vi "MSScript_Exe_MSProcess.vi"(8 "error in (no error)":errorcluster, 9 "EXPR Index in":i32, 11 "MSScript in":refnum<class "MSScript.lvclass">) -> (0 "error out":errorcluster, 1 "EXPR Index out":i32, 3 "MSScript out":refnum<class "MSScript.lvclass">)   [LabVIEW 2018, in "MSScript.lvclass"]
uses:
  MSScript.lvclass
  MSScript.lvclass/MSScript.ctl
  MSScript_Error_(6006)ParamErr.vi
  MSScript_Error_(6002)UndefinedSentence.vi
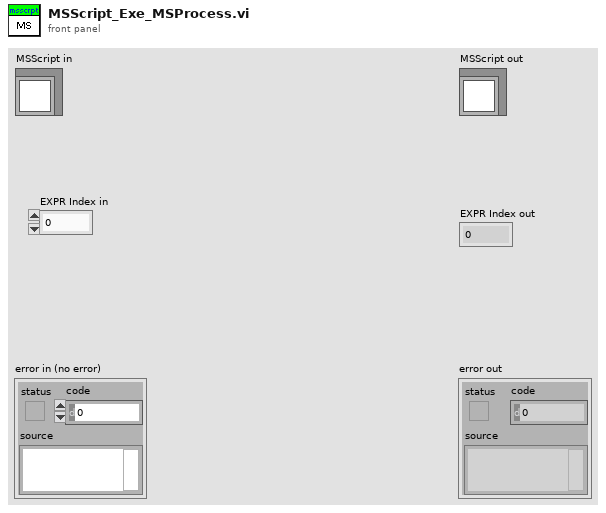
[diagram p1: front panel]
types:
  T1 = cluster{"Colour":u32, "Italic":bool, "Bold":bool}
  T2 = cluster{"Type":string, "NAME":cluster{"STR":string, "Start":i32}, "PARAMs":cluster{"STR":string, "Start":i32}[]}[]
  T3 = cluster{"Type":string, "NAME":cluster{"STR":string, "Start":i32}, "PARAMs":cluster{"STR":string, "Start":i32}[]}
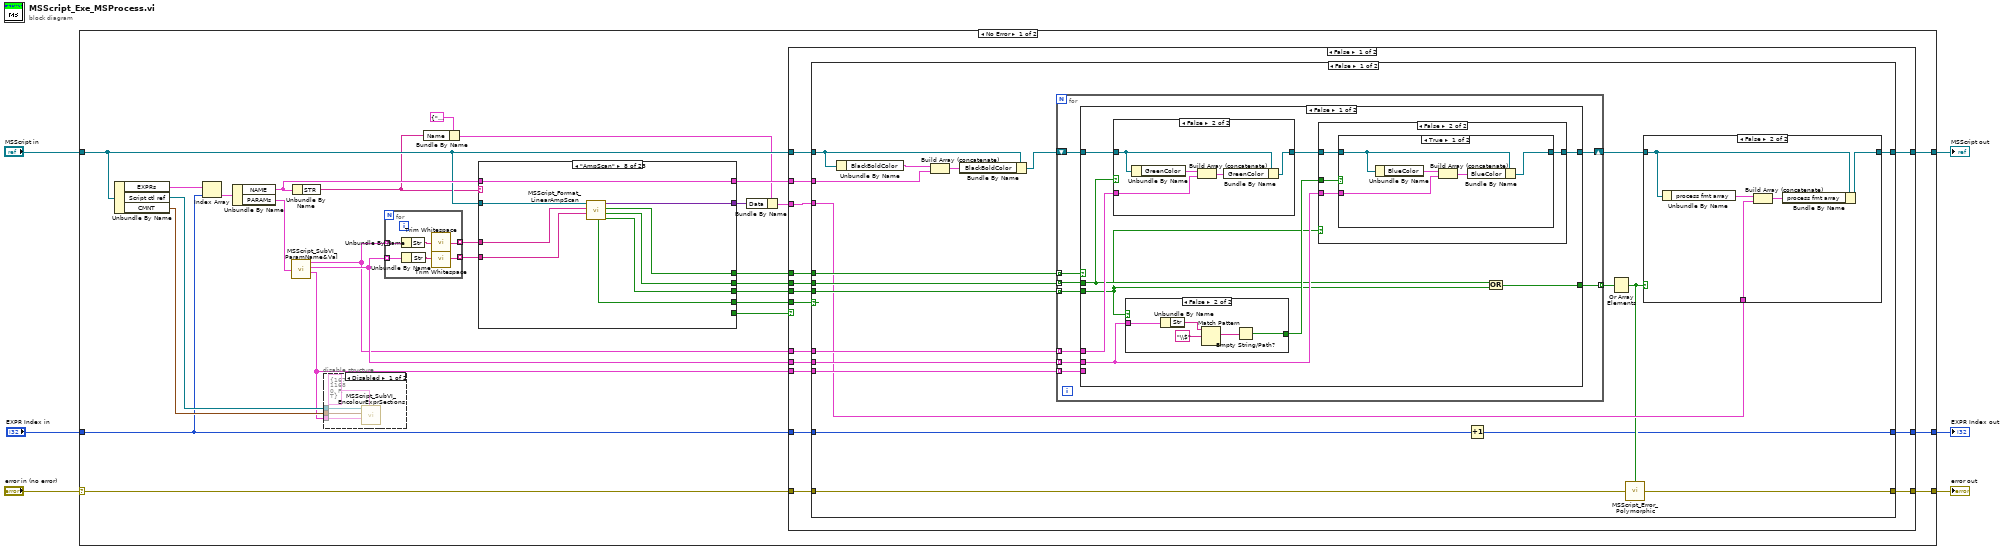
[diagram p0: block diagram]
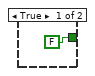
[diagram p3: hidden frame]
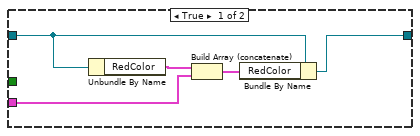
[diagram p4: hidden frame]
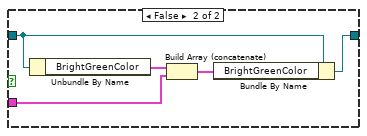
[diagram p5: hidden frame]
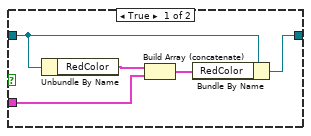
[diagram p6: hidden frame]
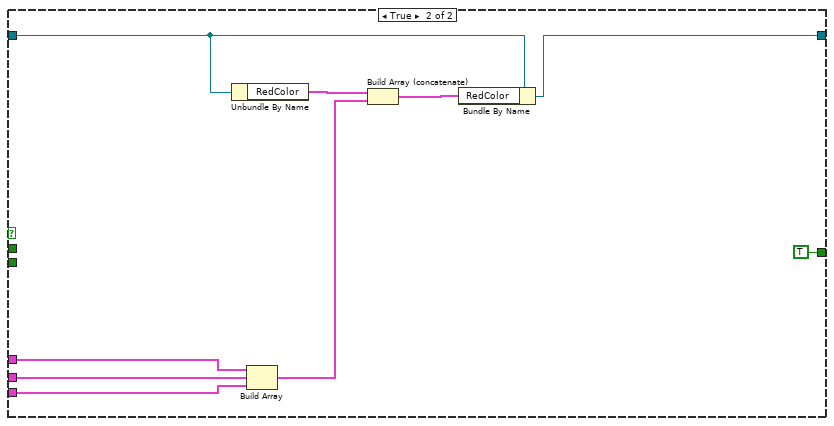
[diagram p7: hidden frame]
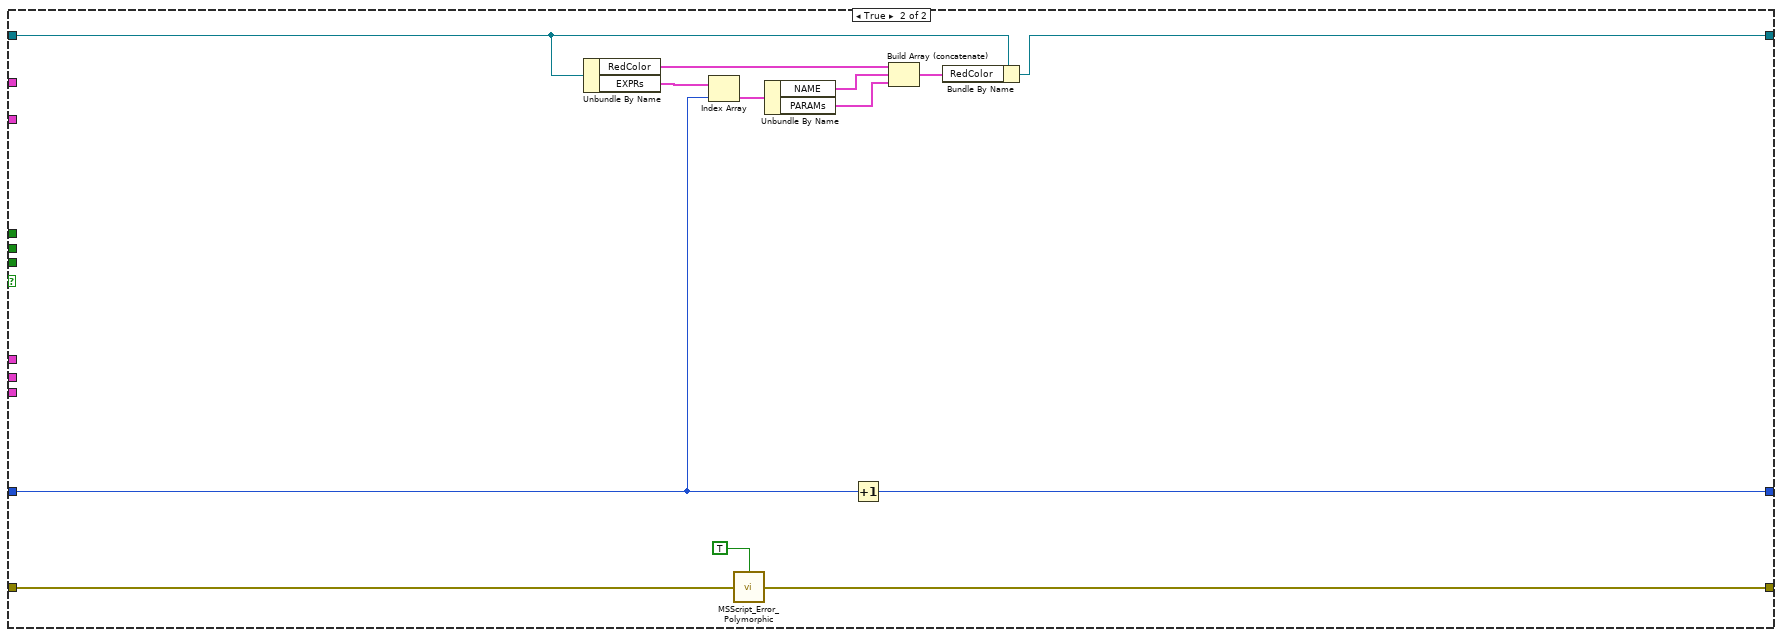
[diagram p8: hidden frame]
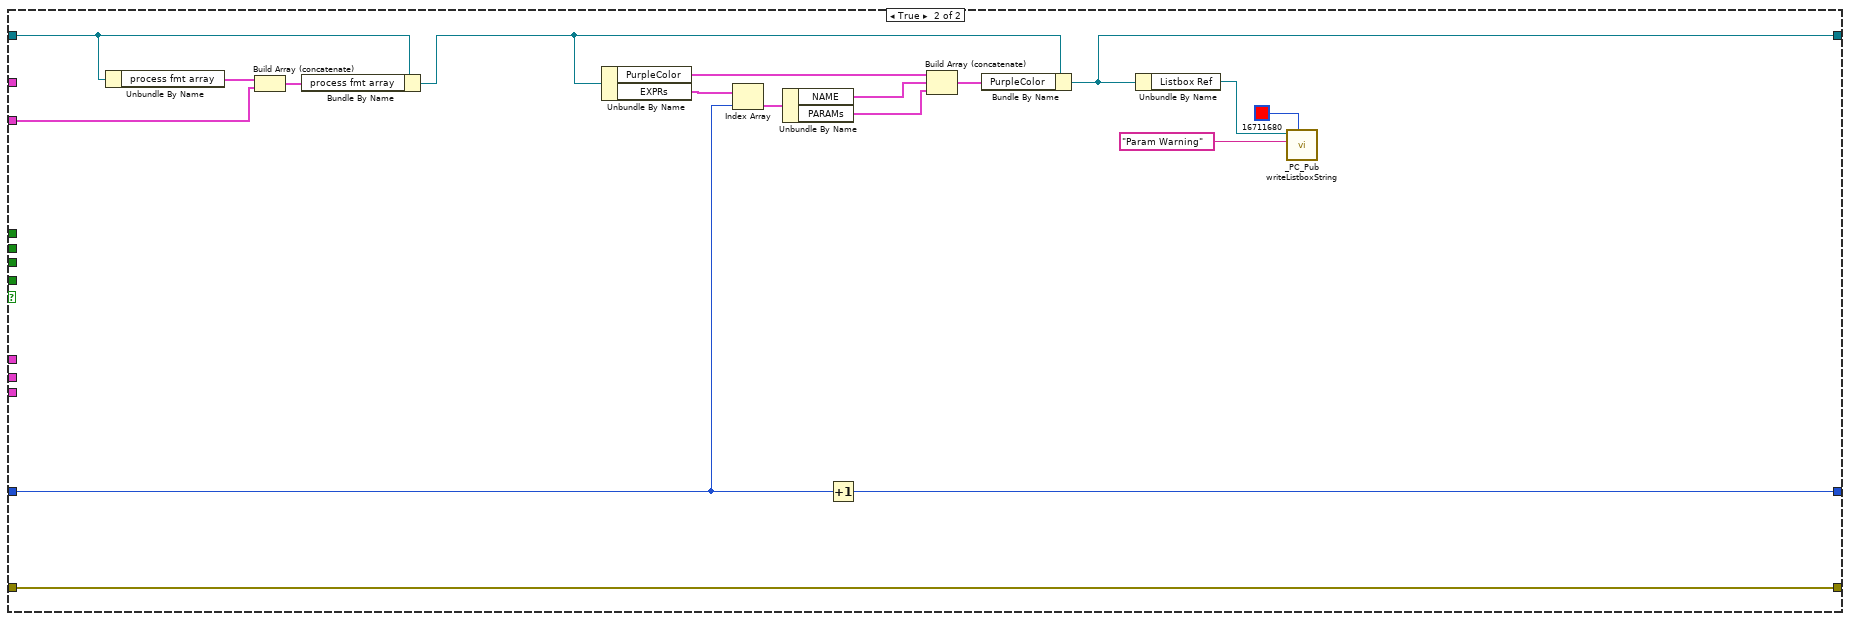
[diagram p9: hidden frame]
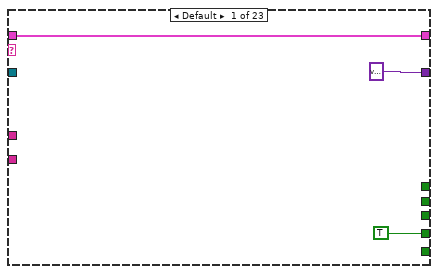
[diagram p11: hidden frame]
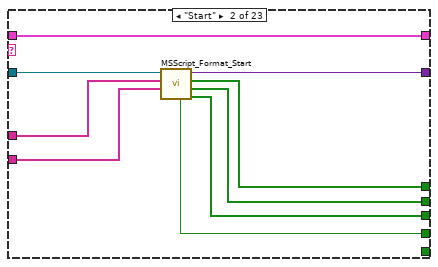
[diagram p12: hidden frame]
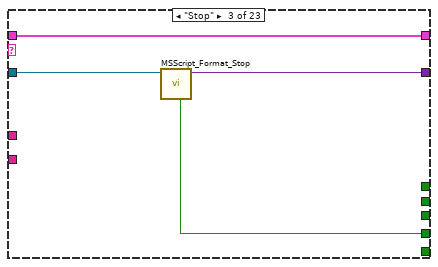
[diagram p13: hidden frame]
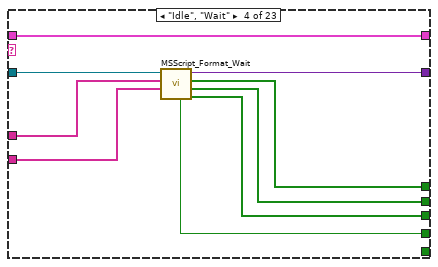
[diagram p14: hidden frame]
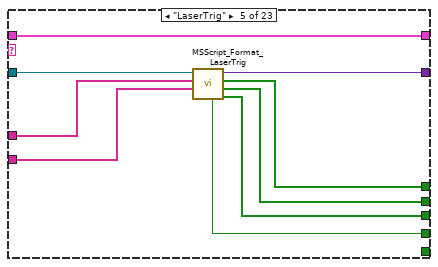
[diagram p15: hidden frame]
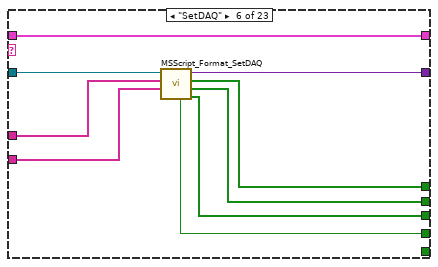
[diagram p16: hidden frame]
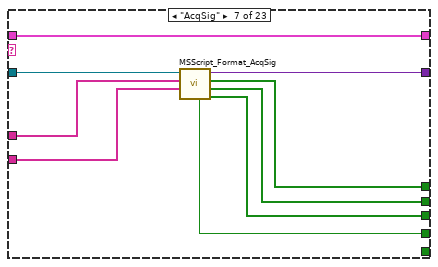
[diagram p17: hidden frame]
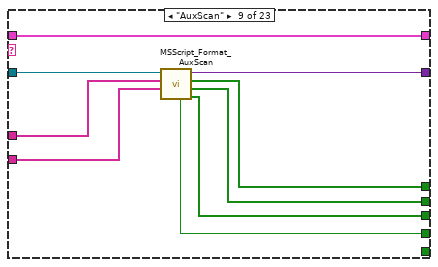
[diagram p18: hidden frame]
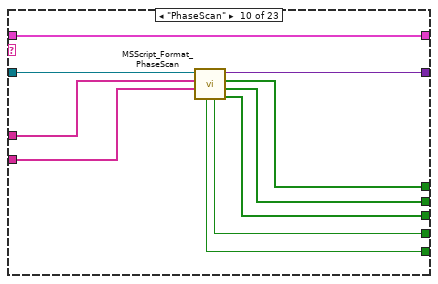
[diagram p19: hidden frame]
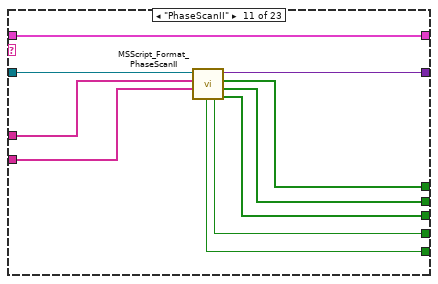
[diagram p20: hidden frame]
diagram:
  n1 = case shown="No Error" "error in (no error)" {
    selector: "error in (no error)" -> [w22 w379]
    tunnel: [w21 w379] -> w5
    tunnel: [w24 w378] -> w3
    tunnel: "MSScript in" -> [w14 w378]
    tunnel: "EXPR Index in" -> [w20 _]
    tunnel: [w16 _] -> w1
    frame No Error {
      n2 = Unbundle By Name(w14) -> ("EXPRs"=w34:T2, "Script ctl ref"=w30:refnum<vi>, "CMNT"=w31:cluster{"Start":u32, "End":u32}[])
      n3 = Index Array(array=w34, index=w20) -> (element=w33:T3)
      n4 = Unbundle By Name(w33) -> ("NAME"=w15:cluster{"STR":string, "Start":i32}, "PARAMs"=w32:cluster{"STR":string, "Start":i32}[])
      n5 = call "MSScript_SubVI_ParamName&Val.vi"("PARAMs"=w32) -> ("PARAM.NAMEs"=w18:cluster{"Str":string, "Start":i32}[], "PARAM.VALs"=w19:cluster{"Str":string, "Start":i32}[], "PARAM.EqualSign"=w17:cluster{"Str":string, "Start":i32}[])  [unwired: 4 in, 1 out]
      n6 = Unbundle By Name(w15) -> ("STR"=w11:string)
      n7 = disable-structure shown="Disabled" {
        disable-tunnel: w31 -> [w172 _]
        disable-tunnel: w30 -> [w171 _]
        disable-tunnel: w17 -> [w170 _]
        frame Disabled {
          n8 = call "MSScript_SubVI_EncolourExprSections.vi"("TextProperties"=T1 {"Colour"=16711680, "Italic"=FALSE, "Bold"=TRUE}, "Expression Sections"=w170, "CMNT"=w172, "String in"=w171) -> ()  [unwired: 7 in, 1 out]
        }
        frame Enabled {
        }
      }
      n9 = for {
        tunnel: w18 -> [w178] mode=indexing
        tunnel: w19 -> [w177] mode=indexing
        tunnel: [w174] -> w29 mode=indexing
        tunnel: [w173] -> w28 mode=indexing
        n10 = Unbundle By Name(w178) -> ("Str"=w176:string)
        n11 = Unbundle By Name(w177) -> ("Str"=w175:string)
        n12 = call <vilib>:"Trim Whitespace.vi"("string"=w176) -> ("trimmed string"=w174:string)  [unwired: 1 in]
        n13 = call <vilib>:"Trim Whitespace.vi"("string"=w175) -> ("trimmed string"=w173:string)  [unwired: 1 in]
      }
      n14 = Bundle By Name(cluster=cluster{"Name":string, "Data":variant} {"Name"="", "Data"=variant} ("process fmt"), "Name"=w11) -> (w9:cluster{"Name":string, "Data":variant})
      n15 = case shown="\"AmpScan\"" w11 {
        tunnel: w29 -> [_ w188 _ w203 w207 w216 w223 w239 w243 w258 w260 w270 w280 w291 w305 w314 w323 w332 w338 w348 w353 w368 w377]
        tunnel: w28 -> [_ w187 _ w202 w208 w215 w222 w238 w242 w257 w261 w271 w281 w290 w304 w313 w322 w331 w337 w347 w352 w367 w376]
        tunnel: [variant w190 w194 w197 w212 w221 w228 w237 w248 w256 w267 w277 w286 w296 w303 w312 w317 w324 w339 w346 w358 w362 w371] -> w8
        tunnel: [_ w189 _ w198 w211 w220 w227 w236 w246 w255 w266 w276 w285 w292 w302 w311 w318 w327 w333 w345 w357 w363 w372] -> w27
        tunnel: [_ w186 _ w199 w210 w219 w226 w235 w245 w254 w265 w275 w284 w293 w301 w310 w319 w328 w334 w344 w356 w364 w373] -> w26
        tunnel: [_ w185 _ w200 w209 w218 w225 w234 w244 w253 w264 w274 w283 w294 w300 w309 w320 w329 w335 w343 w355 w365 w374] -> w25
        tunnel: [TRUE ("#ofParamError") w184 w193 w201 w206 w217 w224 w233 w247 w252 w263 w273 w282 w295 w299 w308 w321 w330 w336 w342 w351 w366 w375] -> w23
        tunnel: w15 -> [w180 w183 w192 w196 w205 w214 w230 w231 w240 w251 w268 w278 w287 w289 w298 w307 w316 w326 w341 w350 w359 w361 w370]
        tunnel: w14 -> [_ w182 w191 w195 w204 w213 w229 w232 w241 w250 w259 w269 w279 w288 w297 w306 w315 w325 w340 w349 w354 w360 w369]
        tunnel: [w180 w183 w192 w196 w205 w214 w230 w231 w240 w251 w268 w278 w287 w289 w298 w307 w316 w326 w341 w350 w359 w361 w370] -> w13
        tunnel: [_ _ _ _ _ _ _ _ _ w249 w262 w272 _ _ _ _ _ _ _ _ _ _ _] -> w7
        frame Default {
        }
        frame "Start" {
          n16 = call "MSScript_Format_Start.vi"("ValueArray"=w187, "TagArray"=w188, "MSScript in"=w182) -> ("ValueErrorArray"=w185:bool[], "TagErrorArray"=w186:bool[], "ParamErrorArray"=w189:bool[], "Data"=w190:variant, "#ofParamError"=w184:bool)  [unwired: 4 in]
        }
        frame "Stop" {
          n17 = call "MSScript_Format_Stop.vi"("MSScript in"=w191) -> ("Data"=w194:variant, "#ofParamError"=w193:bool)  [unwired: 9 in]
        }
        frame "Idle", "Wait" {
          n18 = call "MSScript_Format_Wait.vi"("ValueArray"=w202, "TagArray"=w203, "MSScript in"=w195) -> ("ValueErrorArray"=w200:bool[], "TagErrorArray"=w199:bool[], "ParamErrorArray"=w198:bool[], "Data"=w197:variant, "#ofParamError"=w201:bool)  [unwired: 4 in]
        }
        frame "LaserTrig" {
          n19 = call "MSScript_Format_LaserTrig.vi"("ValueArray"=w208, "TagArray"=w207, "MSScript in"=w204) -> ("ValueErrorArray"=w209:bool[], "TagErrorArray"=w210:bool[], "ParamErrorArray"=w211:bool[], "Data"=w212:variant, "#ofParamError"=w206:bool)  [unwired: 4 in]
        }
        frame "SetDAQ" {
          n20 = call "MSScript_Format_SetDAQ.vi"("ValueArray"=w215, "TagArray"=w216, "MSScript.lvclass"=w213) -> ("ValueErrorArray"=w218:bool[], "TagErrorArray"=w219:bool[], "ParamErrorArray"=w220:bool[], "Data"=w221:variant, "#ofParamError"=w217:bool)  [unwired: 4 in]
        }
        frame "AcqSig" {
          n21 = call "MSScript_Format_AcqSig.vi"("ValueArray"=w222, "TagArray"=w223, "MSScript in"=w229) -> ("ValueErrorArray"=w225:bool[], "TagErrorArray"=w226:bool[], "ParamErrorArray"=w227:bool[], "Data"=w228:variant, "#ofParamError"=w224:bool)  [unwired: 4 in]
        }
        frame "AmpScan" {
          n22 = call "MSScript_Format_LinearAmpScan.vi"("ValueArray"=w238, "NameArray"=w239, "MSScript in"=w232) -> ("ValueErrorArray"=w234:bool[], "TagErrorArray"=w235:bool[], "ParamErrorArray"=w236:bool[], "data out"=w237:variant, "#ofParamError"=w233:bool)  [unwired: 4 in]
        }
        frame "AuxScan" {
          n23 = call "MSScript_Format_AuxScan.vi"("ValueArray"=w242, "TagArray"=w243, "MSScript in"=w241) -> ("ValueErrorArray"=w244:bool[], "TagErrorArray"=w245:bool[], "ParamErrorArray"=w246:bool[], "Data"=w248:variant, "#ofParamError"=w247:bool)  [unwired: 4 in]
        }
        frame "PhaseScan" {
          n24 = call "MSScript_Format_PhaseScan.vi"("ValueArray"=w257, "TagArray"=w258, "MSScript in"=w250) -> ("ValueErrorArray"=w253:bool[], "TagErrorArray"=w254:bool[], "ParamErrorArray"=w255:bool[], "Data"=w256:variant, "#ofParamError"=w252:bool, "Warning?"=w249:bool)  [unwired: 3 in]
        }
        frame "PhaseScanII" {
          n25 = call "MSScript_Format_PhaseScanII.vi"("ValueArray"=w261, "TagArray"=w260, "MSScript in"=w259) -> ("ValueErrorArray"=w264:bool[], "TagErrorArray"=w265:bool[], "ParamErrorArray"=w266:bool[], "Data"=w267:variant, "#ofParamError"=w263:bool, "Warning?"=w262:bool)  [unwired: 3 in]
        }
        frame "CLFreqScan" {
          n26 = call "MSScript_Format_CLFreqScan.vi"("ValueArray"=w271, "TagArray"=w270, "MSScript in"=w269) -> ("ValueErrorArray"=w274:bool[], "TagErrorArray"=w275:bool[], "ParamErrorArray"=w276:bool[], "Data"=w277:variant, "#ofParamError"=w273:bool, "Warning?"=w272:bool)  [unwired: 3 in]
        }
        frame "ResetRFPhase", "RstRFPhase" {
          n27 = call "MSScript_Format_ResetRFPhase.vi"("ValueArray"=w281, "TagArray"=w280, "MSScript.lvclass"=w279) -> ("ValueErrorArray"=w283:bool[], "TagErrorArray"=w284:bool[], "ParamErrorArray"=w285:bool[], "Data"=w286:variant, "#ofParamError"=w282:bool)  [unwired: 4 in]
        }
        frame "UpdConj" {
          n28 = call "MSScript_Format_UpdConj.vi"("ValueArray"=w290, "TagArray"=w291, "MSScript.lvclass"=w288) -> ("ValueErrorArray"=w294:bool[], "TagErrorArray"=w293:bool[], "ParamErrorArray"=w292:bool[], "Data"=w296:variant, "#ofParamError"=w295:bool)  [unwired: 4 in]
        }
        frame "UpdAO" {
          n29 = call "MSScript_Format_UpdAO.vi"("ValueArray"=w304, "TagArray"=w305, "MSScript.lvclass"=w297) -> ("ValueErrorArray"=w300:bool[], "TagErrorArray"=w301:bool[], "ParamErrorArray"=w302:bool[], "Data"=w303:variant, "#ofParamError"=w299:bool)  [unwired: 4 in]
        }
        frame "UpdDO" {
          n30 = call "MSScript_Format_UpdDO.vi"("ValueArray"=w313, "TagArray"=w314, "MSScript.lvclass"=w306) -> ("ValueErrorArray"=w309:bool[], "TagErrorArray"=w310:bool[], "ParamErrorArray"=w311:bool[], "Data"=w312:variant, "#ofParamError"=w308:bool)  [unwired: 4 in]
        }
        frame "UpdIGVolt", "UpdIGVolts" {
          n31 = call "MSScript_Format_UpdIGVolts.vi"("ValueArray"=w322, "TagArray"=w323, "MSScript.lvclass"=w315) -> ("ValueErrorArray"=w320:bool[], "TagErrorArray"=w319:bool[], "ParamErrorArray"=w318:bool[], "Data"=w317:variant, "#ofParamError"=w321:bool)  [unwired: 4 in]
        }
        frame "UpdRFChBias" {
          n32 = call "MSScript_Format_UpdRFChBias.vi"("ValueArray"=w331, "TagArray"=w332, "MSScript.lvclass"=w325) -> ("ValueErrorArray"=w329:bool[], "TagErrorArray"=w328:bool[], "ParamErrorArray"=w327:bool[], "Data"=w324:variant, "#ofParamError"=w330:bool)  [unwired: 4 in]
        }
        frame "UpdRFChFunc" {
          n33 = call "MSScript_Format_UpdRFChFunc.vi"("ValueArray"=w337, "TagArray"=w338, "MSScript.lvclass"=w340) -> ("ValueErrorArray"=w335:bool[], "TagErrorArray"=w334:bool[], "ParamErrorArray"=w333:bool[], "Data"=w339:variant, "#ofParamError"=w336:bool)  [unwired: 4 in]
        }
        frame "UpdRFChScale" {
          n34 = call "MSScript_Format_UpdRFChScale.vi"("ValueArray"=w347, "TagArray"=w348, "MSScript.lvclass"=w349) -> ("ValueErrorArray"=w343:bool[], "TagErrorArray"=w344:bool[], "ParamErrorArray"=w345:bool[], "Data"=w346:variant, "#ofParamError"=w342:bool)  [unwired: 4 in]
        }
        frame "UpdAuxArbPulses" {
          n35 = call "MSScript_Format_UpdAuxArbPulses.vi"("ValueArray"=w352, "TagArray"=w353, "MSScript.lvclass"=w354) -> ("ValueErrorArray"=w355:bool[], "TagErrorArray"=w356:bool[], "ParamErrorArray"=w357:bool[], "Data"=w358:variant, "#ofParamError"=w351:bool)  [unwired: 4 in]
        }
        frame "FGen" {
          n36 = call "MSScript_Format_FGen.vi"("ValueArray"=w367, "TagArray"=w368, "MSScript in"=w360) -> ("ValueErrorArray"=w365:bool[], "TagErrorArray"=w364:bool[], "ParamErrorArray"=w363:bool[], "Data"=w362:variant, "#ofParamError"=w366:bool)  [unwired: 4 in]
        }
        frame "IonGate" {
          n37 = call "MSScript_Format_IonGate.vi"("ValueArray"=w376, "TagArray"=w377, "MSScript in"=w369) -> ("ValueErrorArray"=w374:bool[], "TagErrorArray"=w373:bool[], "ParamErrorArray"=w372:bool[], "Data"=w371:variant, "#ofParamError"=w375:bool)  [unwired: 4 in]
        }
      }
      n38 = Bundle By Name(cluster=w9, "Data"=w8) -> (w10:cluster{"Name":string, "Data":variant})
      n39 = case shown="False" w7 {
        tunnel: w27 -> [w49 _]
        tunnel: w26 -> [w48 _]
        tunnel: w25 -> [w47 _]
        tunnel: [w46 w159] -> w24
        tunnel: w23 -> [w45 _]
        tunnel: w22 -> [w44 w163]
        tunnel: [w43 w163] -> w21
        tunnel: w20 -> [w42 w162]
        tunnel: w19 -> [w41 _]
        tunnel: w18 -> [w40 _]
        tunnel: w17 -> [w39 _]
        tunnel: [w38 w161] -> w16
        tunnel: w14 -> [w37 w152]
        tunnel: w13 -> [w36 _]
        tunnel: w10 -> [w35 w153]
        frame False {
          n40 = case shown="False" w45 {
            tunnel: w49 -> [w69 _]
            tunnel: w48 -> [w68 _]
            tunnel: w47 -> [w67 _]
            tunnel: w37 -> [w52 w142]
            tunnel: w35 -> [w58 _]
            tunnel: [w59 w141] -> w46
            tunnel: w44 -> [w63 w150]
            tunnel: [w62 w149] -> w43
            tunnel: w42 -> [w56 w140]
            tunnel: w41 -> [w66 _]
            tunnel: w40 -> [w65 _]
            tunnel: w39 -> [w64 _]
            tunnel: [w55 w139] -> w38
            tunnel: w36 -> [w50 _]
            frame False {
              n41 = Unbundle By Name(w52) -> ("BlackBoldColor"=w54:cluster{"STR":string, "Start":i32}[])
              n42 = Build Array (concatenate)(w54, w50) -> (w53:cluster{"STR":string, "Start":i32}[])
              n43 = Bundle By Name(cluster=w52, "BlackBoldColor"=w53) -> (w51:refnum<class "MSScript.lvclass">)
              n44 = for {
                tunnel: w69 -> [w84] mode=indexing
                tunnel: w65 -> [w83] mode=indexing
                tunnel: w66 -> [w82] mode=indexing
                tunnel: w64 -> [w81] mode=indexing
                tunnel: w68 -> [w78] mode=indexing
                tunnel: w67 -> [w77] mode=indexing
                shift-right: [w79] -> w60
                shift-left: w51 -> [w80]
                tunnel: [w76] -> w61 mode=indexing
                n45 = case shown="False" w84 {
                  tunnel: w83 -> [w92 w137]
                  tunnel: w82 -> [w89 w136]
                  tunnel: w81 -> [_ w135]
                  tunnel: w80 -> [w93 w133]
                  tunnel: [w90 w134] -> w79
                  tunnel: w78 -> [w87 _]
                  tunnel: w77 -> [w86 _]
                  tunnel: [w85 TRUE] -> w76
                  frame False {
                    n46 = case shown="False" w87 {
                      tunnel: w93 -> [w123 w128]
                      tunnel: [w122 w127] -> w91
                      tunnel: w92 -> [w120 w125]
                      frame True {
                        n47 = Unbundle By Name(w123) -> ("RedColor"=w121:cluster{"STR":string, "Start":i32}[])
                        n48 = Build Array (concatenate)(w121, w120) -> (w119:cluster{"Str":string, "Start":i32}[])
                        n49 = Bundle By Name(cluster=w123, "RedColor"=w119) -> (w122:refnum<class "MSScript.lvclass">)
                      }
                      frame False {
                        n50 = Unbundle By Name(w128) -> ("GreenColor"=w126:cluster{"STR":string, "Start":i32}[])
                        n51 = Build Array (concatenate)(w126, w125) -> (w124:cluster{"Str":string, "Start":i32}[])
                        n52 = Bundle By Name(cluster=w128, "GreenColor"=w124) -> (w127:refnum<class "MSScript.lvclass">)
                      }
                    }
                    n53 = case shown="False" w86 {
                      tunnel: w89 -> [_ w97]
                      tunnel: [FALSE w95] -> w88
                      frame True {
                      }
                      frame False {
                        n54 = Unbundle By Name(w97) -> ("Str"=w98:string)
                        n55 = Match Pattern(string=w98, regular expression="\\$") -> (match substring=w96:string)  [unwired: 1 in, 3 out]
                        n56 = Empty String/Path?(string/path=w96) -> (empty?=w95:bool)
                      }
                    }
                    n57 = case shown="False" w86 {
                      tunnel: w91 -> [w100 w108]
                      tunnel: [w104 w107] -> w90
                      tunnel: w89 -> [w102 w106]
                      tunnel: w88 -> [_ w105]
                      frame True {
                        n58 = Unbundle By Name(w100) -> ("RedColor"=w103:cluster{"STR":string, "Start":i32}[])
                        n59 = Build Array (concatenate)(w103, w102) -> (w101:cluster{"Str":string, "Start":i32}[])
                        n60 = Bundle By Name(cluster=w100, "RedColor"=w101) -> (w104:refnum<class "MSScript.lvclass">)
                      }
                      frame False {
                        n61 = case shown="True" w105 {
                          tunnel: w108 -> [w113 w118]
                          tunnel: [w112 w117] -> w107
                          tunnel: w106 -> [w109 w114]
                          frame True {
                            n62 = Unbundle By Name(w113) -> ("BlueColor"=w111:cluster{"STR":string, "Start":i32}[])
                            n63 = Build Array (concatenate)(w111, w109) -> (w110:cluster{"Str":string, "Start":i32}[])
                            n64 = Bundle By Name(cluster=w113, "BlueColor"=w110) -> (w112:refnum<class "MSScript.lvclass">)
                          }
                          frame False {
                            n65 = Unbundle By Name(w118) -> ("BrightGreenColor"=w116:cluster{"STR":string, "Start":i32}[])
                            n66 = Build Array (concatenate)(w116, w114) -> (w115:cluster{"Str":string, "Start":i32}[])
                            n67 = Bundle By Name(cluster=w118, "BrightGreenColor"=w115) -> (w117:refnum<class "MSScript.lvclass">)
                          }
                        }
                      }
                    }
                    n68 = Or(x=w87, y=w86) -> (x .or. y?=w85:bool)
                  }
                  frame True {
                    n69 = Unbundle By Name(w133) -> ("RedColor"=w132:cluster{"STR":string, "Start":i32}[])
                    n70 = Build Array(w137, w136, w135) -> (w131:cluster{"Str":string, "Start":i32}[])
                    n71 = Build Array (concatenate)(w132, w131) -> (w130:cluster{"Str":string, "Start":i32}[])
                    n72 = Bundle By Name(cluster=w133, "RedColor"=w130) -> (w134:refnum<class "MSScript.lvclass">)
                  }
                }
              }
              n73 = Increment(x=w56) -> (x+1=w55:i32)
              n74 = Or Array Elements(Boolean array=w61) -> (logical OR=w57:bool)
              n75 = call-poly "MSScript_Error_Polymorphic.vi"("error in (no error)"=w63, "ErrBoolean"=w57) -> ("error out"=w62:errorcluster)
              n76 = case shown="False" w57 {
                tunnel: w60 -> [w70 w73]
                tunnel: [w70 w72] -> w59
                tunnel: w58 -> [_ w71]
                frame True {
                }
                frame False {
                  n77 = Unbundle By Name(w73) -> ("process fmt array"=w74:cluster{"Name":string, "Data":variant}[])
                  n78 = Build Array (concatenate)(w74, w71) -> (w75:cluster{"Name":string, "Data":variant}[])
                  n79 = Bundle By Name(cluster=w73, "process fmt array"=w75) -> (w72:refnum<class "MSScript.lvclass">)
                }
              }
            }
            frame True {
              n80 = Unbundle By Name(w142) -> ("RedColor"=w143:cluster{"STR":string, "Start":i32}[], "EXPRs"=w147:T2)
              n81 = Index Array(array=w147, index=w140) -> (element=w148:T3)
              n82 = call-poly "MSScript_Error_Polymorphic.vi"("error in (no error)"=w150, "ErrBoolean"=TRUE) -> ("error out"=w149:errorcluster)
              n83 = Unbundle By Name(w148) -> ("NAME"=w144:cluster{"STR":string, "Start":i32}, "PARAMs"=w138:cluster{"STR":string, "Start":i32}[])
              n84 = Increment(x=w140) -> (x+1=w139:i32)
              n85 = Build Array (concatenate)(w143, w144, w138) -> (w146:cluster{"STR":string, "Start":i32}[])
              n86 = Bundle By Name(cluster=w142, "RedColor"=w146) -> (w141:refnum<class "MSScript.lvclass">)
            }
          }
        }
        frame True {
          n87 = Unbundle By Name(w152) -> ("process fmt array"=w154:cluster{"Name":string, "Data":variant}[])
          n88 = Build Array (concatenate)(w154, w153) -> (w155:cluster{"Name":string, "Data":variant}[])
          n89 = Bundle By Name(cluster=w152, "process fmt array"=w155) -> (w151:refnum<class "MSScript.lvclass">)
          n90 = Unbundle By Name(w151) -> ("PurpleColor"=w164:cluster{"STR":string, "Start":i32}[], "EXPRs"=w167:T2)
          n91 = Index Array(array=w167, index=w162) -> (element=w168:T3)
          n92 = Unbundle By Name(w168) -> ("NAME"=w165:cluster{"STR":string, "Start":i32}, "PARAMs"=w160:cluster{"STR":string, "Start":i32}[])
          n93 = Increment(x=w162) -> (x+1=w161:i32)
          n94 = Build Array (concatenate)(w164, w165, w160) -> (w166:cluster{"STR":string, "Start":i32}[])
          n95 = Bundle By Name(cluster=w151, "PurpleColor"=w166) -> (w159:refnum<class "MSScript.lvclass">)
          n96 = Unbundle By Name(w159) -> ("Listbox Ref"=w158:refnum<vi>)
          n97 = call "_PC_Pub writeListboxString.vi"("String Color"=u32 16711680, "update_Str"="Param Warning", "Listbox Ref Input"=w158) -> ()  [unwired: 7 in, 2 out]
        }
      }
    }
    frame Error {
    }
  }
  "error out" <- w5
  "MSScript out" <- w3
  "EXPR Index out" <- w1
